vi "Test Set GPIOA0 and GPIOA1.vi"(11 "Test Case In":refnum<class "MCP23017 Test.lvclass">) -> (0 "error out":errorcluster, 3 "Test Case Out":refnum<class "MCP23017 Test.lvclass">)   [LabVIEW 2020, in "MCP23017 Test.lvclass"]
uses:
  MCP23017 Test.lvclass
  C:/Program Files (x86)/National Instruments/LabVIEW 2020/vi.lib/Astemes/LUnit/Test Case.lvclass
  source/GPIO Channel.ctl
  Mock I2C Bus/Mock I2C Bus.lvclass
  C:/Program Files (x86)/National Instruments/LabVIEW 2020/vi.lib/Astemes/LMock/Mock.lvclass
  C:/git/astemes-mocking-exercise/source/I2C Bus Interface/I2C Bus.lvclass
  <vilib>/Astemes/LMock/One Identical Inputs.vi
  <vilib>/Astemes/LMock/LMock Verifier.lvclass
  <vilib>/Astemes/LMock/LMock.lvlib
  C:/git/astemes-mocking-exercise/tests/Mock I2C Bus/Mock I2C Bus.lvclass
  source/MCP23017/MCP23017.lvclass
  <vilib>/Astemes/LMock/LMock One.lvlib
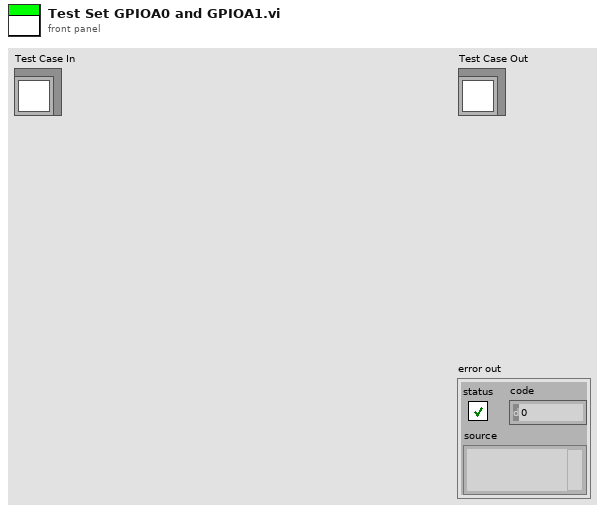
[diagram p1: front panel]
types:
  T1 = typedef "MCP23017.lvclass/GPIO Channel.ctl" = enum16{"GPA.0", "GPA.1", "GPA.2", "GPA.3", "GPA.4", "GPA.5", "GPA.6", "GPA.7", "GPB.0", "GPB.1", "GPB.2", "GPB.3", "GPB.4", "GPB.5", "GPB.6", "GPB.7"}
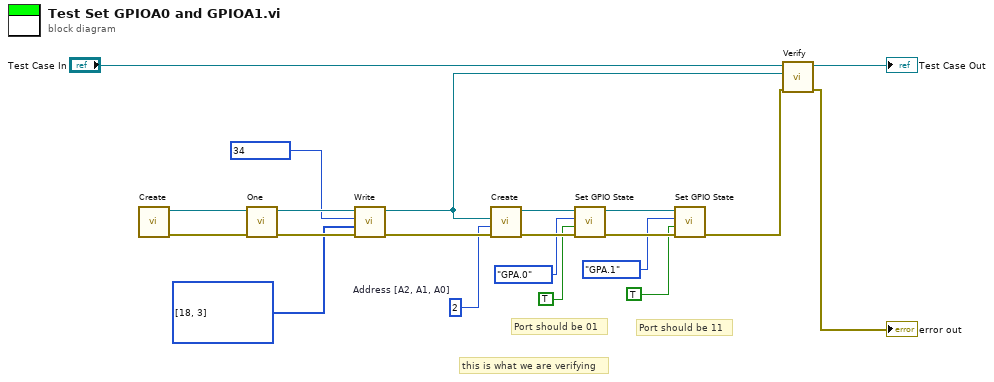
[diagram p0: block diagram]
diagram:
  w9 = u8 2  # Address [A2, A1, A0]
  # "this is what we are verifying"
  # "this is what we are verifying"
  # "Port should be 11"
  # "Port should be 01"
  n1 = call "Create.vi"() -> ("error out"=w18:errorcluster, "Mock Class Generator out"=w16:refnum<class "Mock I2C Bus.lvclass">)  [unwired: 10 in]
  n2 = call-poly <vilib>:"One.vi"("error in (no error)"=w18, "Mock in"=w16) -> ("error out"=w17:errorcluster, "Mock out"=w15:refnum<class "Mock I2C Bus.lvclass">)  [unwired: 8 in]
  n3 = call-dynamic "Write.vi"("error in (no error)"=w17, "Data"=u8[] [18, 3], "Address"=u8 34, "I2C Bus In"=w15) -> ("error out"=w12:errorcluster, "I2C Bus Out"=w10:refnum<class "Mock I2C Bus.lvclass">)  [unwired: 6 in]
  n4 = call "Create.vi"("error in (no error)"=w12, "Address [A2, A1, A0]"=w9, "I2C Bus"=w10) -> ("error out"=w11:errorcluster, "MCP23017"=w7:refnum<class "MCP23017.lvclass">)  [unwired: 7 in]
  n5 = call "Set GPIO State.vi"("error in (no error)"=w11, "State"=TRUE, "Channel"=GPIO_Channel."GPA.0", "MCP23017 In"=w7) -> ("error out"=w8:errorcluster, "MCP23017 Out"=w3:refnum<class "MCP23017.lvclass">)  [unwired: 6 in]
  n6 = call "Set GPIO State.vi"("error in (no error)"=w8, "State"=TRUE, "Channel"=GPIO_Channel."GPA.1", "MCP23017 In"=w3) -> ("error out"=w4:errorcluster)  [unwired: 6 in, 1 out]
  n7 = call <vilib>:"Verify.vi"("error in (no error)"=w4, "Mock"=w10, "LUnit Test Case In"="Test Case In") -> ("error out"=→"error out":errorcluster, "LUnit Test Case Out"=→"Test Case Out":refnum<class "MCP23017 Test.lvclass">)  [unwired: 7 in]
